vi "ECOG-About Box.vi"(2 "Parent VI":refnum<vi>) -> ()   [LabVIEW 2020]
uses:
  <vilib>/Platform/browser.llb/Open URL in Default Browser (path).vi
panel:
  in  "link":bool
  in  "OK Button":bool
  out "Version":string
  # "ECOG Monitor"
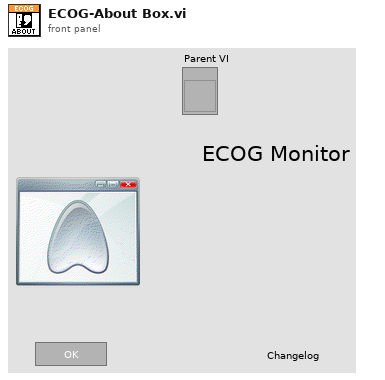
[diagram p1: front panel]
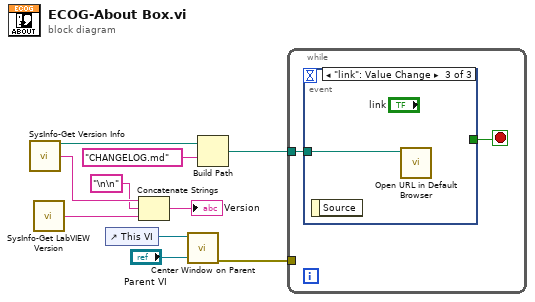
[diagram p0: block diagram]
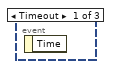
[diagram p2: hidden frame]
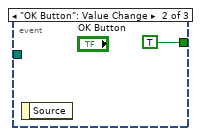
[diagram p3: hidden frame]
diagram:
  n1 = call "SysInfo-Get Version Info.vi"() -> ("folder"=w6:path, "formatted version"=w4:string)  [unwired: 13 in, 1 out]
  n2 = call "SysInfo-Get LabVIEW Version.vi"() -> ("Version Info"=w2:string)  [unwired: 15 in]
  n3 = control-ref of="This VI"() -> (w9:refnum<vi>)
  n4 = Concatenate Strings(w4, "\n\n", w2) -> (→"Version":string)
  n5 = call "Center Window on Parent.vi"("Parent VI"="Parent VI", "VI in"=w9) -> ("error out"=w3:errorcluster)  [unwired: 8 in, 1 out]
  n6 = Build Path(base path=w6, name or relative path="CHANGELOG.md") -> (appended path=w5:path)
  n7 = while {
    tunnel: w5 -> [w11]
    tunnel: w3 -> [_]
    stop <- w12 stop-if-true
    n8 = event shown="[2] \"link\": Value Change" {
      selector: _ -> [_ _ _]
      dyn-events: _ -> [_ _ _]
      timeout: _ -> [_ _ _]
      tunnel: [_ TRUE _] -> w12
      tunnel: w11 -> [_ _ w14]
      event Timeout {
        n9 = event-data() -> ()  [unwired: 1 in, 1 out]
      }
      event "OK Button": Value Change {
        n10 = event-data() -> ()  [unwired: 1 in, 1 out]
      }
      event "link": Value Change {
        n11 = event-data() -> ()  [unwired: 1 in, 1 out]
        n12 = call-poly <vilib>:"Open URL in Default Browser.vi"("path"=w14) -> ()  [unwired: 5 in, 2 out]
      }
    }
  }
